vi "Test Red-y Pressure Control CFG2.vi"(11 "Test Case In":refnum<class "Test Red-y Pressure Control CFG.lvclass">) -> (0 "error out":errorcluster, 3 "Test Case Out":refnum<class "Test Red-y Pressure Control CFG.lvclass">)   [LabVIEW 2024, in "Test Red-y Pressure Control CFG.lvclass"]
uses:
  Test Red-y Pressure Control CFG.lvclass
  C:/Program Files/National Instruments/LabVIEW 2024/vi.lib/Astemes/LUnit/Test Case.lvclass
  Configurations/Pressure Control CFG/Red-y Pressure Control CFG.lvclass
  D:/git/HAL/HAL/Configurations/CFG JSON/CFG JSON.lvclass
  Configurations/Pressure Control CFG/Read Write PE Input.ctl
  <userlib>/_OpenG.lib/lvdata/lvdata.llb/Type Descriptor Enumeration__ogtk.ctl
  <vilib>/Astemes/LUnit/Test Case.lvclass/Test Case.ctl
  <vilib>/Astemes/LUnit/Append Pass Result.vi
  <vilib>/Astemes/LUnit/Append Fail Result.vi
  <vilib>/Astemes/LUnit/Run In UI.vi
  <vilib>/Utility/error.llb/Clear Errors.vi
  <userlib>/_OpenG.lib/lvdata/lvdata.llb/openg_variant.lvlib
  <vilib>/Astemes/LUnit/Test Case.lvclass
  Configurations/CFG JSON/CFG JSON.lvclass
panel:
  in  "setpoint":sgl min=0 max=3 step=0.05 format="%#_g bar ü"
  out "pressure":variant
  in  "stop":bool
  out "flow":variant
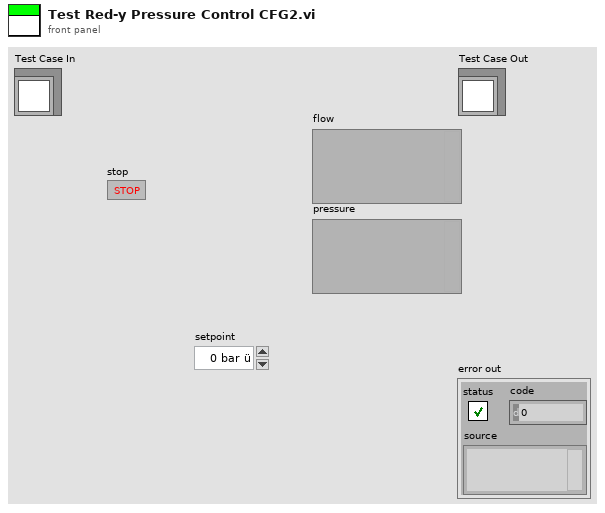
[diagram p1: front panel]
types:
  T1 = typedef "openg_variant.lvlib/Type Descriptor Enumeration__ogtk.ctl" = enum8{"<Null>", "I8", "I16", "I32", "I64", "U8", "U16", "U32", "U64", "SGL", "DBL", "EXT", "CSG", "CDB", "CXT", "0x0F", "0x10", "0x11", "0x12", "0x13", "0x14", "Enum U8", "Enum U16", "Enum U32", "Enum U64", "SGL PQ", "DBL PQ", "EXT PQ", "CSG PQ", "CDB PQ", "CXT PQ", "0x1F", "0x20", "Boolean", "0x22", "0x23", "0x24", "0x25", "0x26", "0x27", "0x28", "0x29", "0x2A", "0x2B", "0x2C", "0x2D", "0x2E", "0x2F", "String", "0x31", "Path", "Pict", "0x34", "0x35", "0x36", "DAQ", "0x38", "0x39", "0x3A", "0x3B", "0x3C", "0x3D", "0x3E", "0x3F", "Array", "0x41", "0x42", "0x43", "0x44", "0x45", "0x46", "0x47", "0x48", "0x49", "0x4A", "0x4B", "0x4C", "0x4D", "0x4E", "0x4F", "Cluster", "0x51", "0x52", "Variant", "Waveform", "0x55", "0x56", "0x57", "0x58", "0x59", "0x5A", "0x5B", "0x5C", "0x5D", "0x5E", "Fixed Point", "0x60", "0x61", "0x62", "0x63", "0x64", "0x65", "0x66", "0x67", "0x68", "0x69", "0x6A", "0x6B", "0x6C", "0x6D", "0x6E", "0x6F", "Refnum", "0x71", "0x72", "Set Collection", "Map Collection"}
  T2 = typedef "Read Write PE Input.ctl" = cluster{"Action":enum16{"Write", "Read"}, "Register":u16, "Type":T1, "Data":variant}
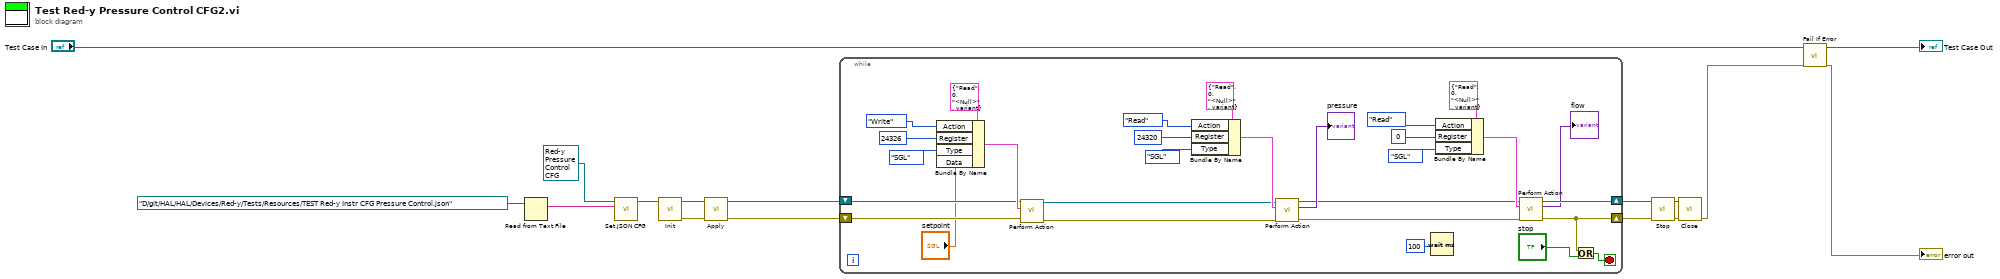
[diagram p0: block diagram]
diagram:
  n1 = Read from Text File(file (use dialog)=path "D:/git/HAL/HAL/Devices/Red-y/Tests/Resources/TEST Red-y Instr CFG Pressure Control.json") -> (text=w5:string)  [unwired: 3 in, 3 out]
  n2 = call "Set JSON CFG.vi"("<JSON> CFG"=w5, "CFG JSON in"=refnum<class "Red-y Pressure Control CFG.lvclass"> refnum ("CFG Base in")) -> ("CFG JSON out"=w12:refnum<class "Red-y Pressure Control CFG.lvclass">)  [unwired: 9 in]
  n3 = call-dynamic "Init.vi"("CFG Base in"=w12) -> ("error out"=w3:errorcluster, "CFG Base out"=w4:refnum<class "Red-y Pressure Control CFG.lvclass">)  [unwired: 9 in]
  n4 = call-dynamic "Apply.vi"("error in"=w3, "Red-y Read Write CFG in"=w4) -> ("error out"=w1:errorcluster, "Red-y Read Write CFG out"=w2:refnum<class "Red-y Pressure Control CFG.lvclass">)  [unwired: 8 in]
  n5 = while {
    shift-right: [w35] -> w9
    shift-left: w1 -> [w19]
    shift-right: [w45] -> w8
    shift-left: w2 -> [w21]
    stop <- w36 stop-if-true
    n6 = Bundle By Name(cluster=T2 {"Action"=enum."Read", "Register"=0, "Type"=enum."<Null>", "Data"=variant}, "Action"=enum16{"Write", "Read"}."Write", "Register"=u16 24326 ("Register Start Address"), "Type"=Type_Descriptor_Enumeration__ogtk."SGL", "Data"="setpoint") -> (w24:T2)
    n7 = call-dynamic "Perform Action.vi"("error in"=w19, "Input"=w24, "Red-y Read Write CFG in"=w21) -> ("error out"=w18:errorcluster, "Red-y Read Write CFG out"=w20:refnum<class "Red-y Pressure Control CFG.lvclass">)  [unwired: 6 in, 1 out]
    n8 = Bundle By Name(cluster=T2 {"Action"=enum."Read", "Register"=0, "Type"=enum."<Null>", "Data"=variant}, "Action"=enum16{"Write", "Read"}."Read", "Register"=u16 24320 ("Register Start Address"), "Type"=Type_Descriptor_Enumeration__ogtk."SGL") -> (w31:T2)
    n9 = call-dynamic "Perform Action.vi"("error in"=w18, "Input"=w31, "Red-y Read Write CFG in"=w20) -> ("error out"=w28:errorcluster, "Output"=→"pressure":variant, "Red-y Read Write CFG out"=w29:refnum<class "Red-y Pressure Control CFG.lvclass">)  [unwired: 6 in]
    n10 = Wait (ms)(milliseconds to wait=u32 100) -> ()  [unwired: 1 out]
    n11 = Bundle By Name(cluster=T2 {"Action"=enum."Read", "Register"=0, "Type"=enum."<Null>", "Data"=variant}, "Action"=enum16{"Write", "Read"}."Read", "Register"=u16 0 ("Register Start Address"), "Type"=Type_Descriptor_Enumeration__ogtk."SGL") -> (w43:T2)
    n12 = call-dynamic "Perform Action.vi"("error in"=w28, "Input"=w43, "Red-y Read Write CFG in"=w29) -> ("error out"=w35:errorcluster, "Output"=→"flow":variant, "Red-y Read Write CFG out"=w45:refnum<class "Red-y Pressure Control CFG.lvclass">)  [unwired: 6 in]
    n13 = Or(x=w35, y="stop") -> (x .or. y?=w36:bool)
  }
  n14 = call-dynamic "Stop.vi"("error in"=w9, "Red-y Read Write CFG in"=w8) -> ("error out"=w11:errorcluster, "Red-y Read Write CFG out"=w10:refnum<class "Red-y Pressure Control CFG.lvclass">)  [unwired: 8 in]
  n15 = call-dynamic "Close.vi"("error in"=w11, "Red-y Read Write CFG in"=w10) -> ("error out"=w7:errorcluster)  [unwired: 8 in, 1 out]
  n16 = call <vilib>:"Fail If Error.vi"("error in (no error)"=w7, "LUnit Test Case In"="Test Case In") -> ("error out"=→"error out":errorcluster, "LUnit Test Case Out"=→"Test Case Out":refnum<class "Test Red-y Pressure Control CFG.lvclass">)  [unwired: 8 in]
